vi "Advanced Serial Write and Read.vi"(4 "stop":bool, 5 "timeout (ms)":u32, 6 "baud rate":u32, 7 "VISA resource name":refnum<visa-resource-name>) -> (1 "gecorr. hoek":string, 2 "afstand":string, 3 "gecorrigeerde afstand":string)   [LabVIEW 8.6]
doc: "The Advanced Serial Read and Write example performs a Serial Port Read, a Serial Port Write, or a combination of these actions while setting some advanced serial features like buffer size, termination characters, and XON/XOFF flow control. The user selects the actions (read or write) on the front panel. If both are selected, the VI will write the data first, read the data and then close the VISA session that is opened to the port. \n\nThe parameters set for the serial port must match the parameters of the connected instrument or device. In this example, the bytes to read parameter specifies the number of bytes that the serial port reads. If there were more bytes at the port than the number specified in bytes to read, those bytes would not be read. Also, if you specify to read more bytes than the number of bytes actually read, you might receive a timeout error message.\n\nINSTRUCTIONS:\n1) Select the serial resource and configuration parameters (baud rate, data bits, parity, stop bits, flow control).\n2) Termination character can be enabled and set. Also, set the required input buffer size prior to running the example.\n3) Select the operations to be performed. \n4) Connect the serial port to your device. If no device is available, perform a loopback test by doing one of the following. Short pins 2 and 3 on a RS-232 cable or short pin 4 to pin 8 and pin 5 to pin 9 on a RS-485/422 cable. \n5) Run the VI to see the data read. (The \"read string\" will match the \"string to write\" if a loopback test was performed.)\n\nThis example exposes several advanced features that you may need for your application. Not all applications need all the features shown in this example. The input buffer size is likely an important setting that you want to control in your application. This example expands upon the flow control option for XON and XOFF, allowing the user to choose those control characters. The timeout parameter has been brought to the front panel so a user can specify the time period the VISA Read will wait for the number of bytes to read before timing out. Also, the user has several controls for the termination character, which is discussed later.\n\nNote that you can press the write and read buttons and change the bytes to read parameters on the fly, while the example is running. However, you must stop the example to change the other configuration parameters after the example has started running, and then run again.\n\nSet the I/O buffer size slightly higher the amount of data you expect to receive. This is very important for applications that don't use flow control, as you may lose characters if the receive buffer overflows.\n\nSetting the timeout period ensures that the operation returns with a timeout error if the operation cannot be performed in the specified time period. \n\nSome devices require a termination character in order to identify the end of command strings. Some devices send a termination character to signify the end of data to be read. \n\nThis example shows how you can end the Read operation once a termination character is detected in the buffer and/or append a termination character at the end of the Write data. To enable the Read to end on a termination character, use the VISA Configure Serial Port or use the VISA Properties Serial End Mode for Reads, Termination Character Enable, and Termination Character. To end the Write with a termination character, use the VISA Properties Serial End Mode for Writes, the Send End Enable, and Termination Character. In this example, the same termination character is used for both the Read and the Write. You can specify two different characters for your application, if desired.\n\nYour application may require specific characters for the XON/XOFF Flow Control. You can specify these characters with the VISA Properties Flow Control XOFF Character and Flow Control XON Character. Note that if the standard XON and XOFF characters are used, then decimal 17 and 19 are unavailable for data values. Remember that using flow control and setting an adequate buffer size allow you to prevent buffer overflows."
uses:
  <vilib>/Instr/_visa.llb/VISA Configure Serial Port (Instr).vi
panel:
  out "current time":timestamp
  out "current GPS time":timestamp
  in  "correctie voor hoek":dbl
  out "gemeten hoek":string
  out "concatenated string":string
  out "actual bytes read":u32
  in  "read":bool
  in  "bytes to read":u32
  out "read string":string
  in  "flow control":u16(ring) items=["None", "XON/XOFF", "RTS/CTS", "DTR/DSR"]
  in  "End write with termination character?":bool
  in  "Input\nbuffer size":u32
  in  "XOFF Character":u8 format="%.0x"
  in  "XON Character":u8 format="%.0x"
  in  "termination char\n(0xA = '\\n' = LF)":u8 format="%.0x"
  in  "End read on termination character?":bool
  in  "parity":u16(ring) items=["None", "Odd", "Even", "Mark", "Space"]
  in  "data bits":u16
  in  "stop bits":u16(ring) items=["1.0", "1.5", "2.0"]
  in  "write":bool
  in  "string to write":string
  # "On Windows/Linux, consider using the Instrument Driver Finder (Help>>Find Instrument Drivers) to search for an instrument driver for your instrument."
  # "Select the serial resource and the operations to be performed.  If all are selected, the VI will write the data first, read data and then close the VISA session that is opened to the port.  This VI will wait until the specified number of bytes is received at the port, until the timeout period is met, or until a termination character is received.  The default termination character in this example is the Line Feed ( ASCII 0xA, '\\n' ).  Also, set the required input buffer size prior to running the example.\nNote: The example loops until the STOP button is pressed."
  # "For additional information select File >> VI Properties >> Documentation"
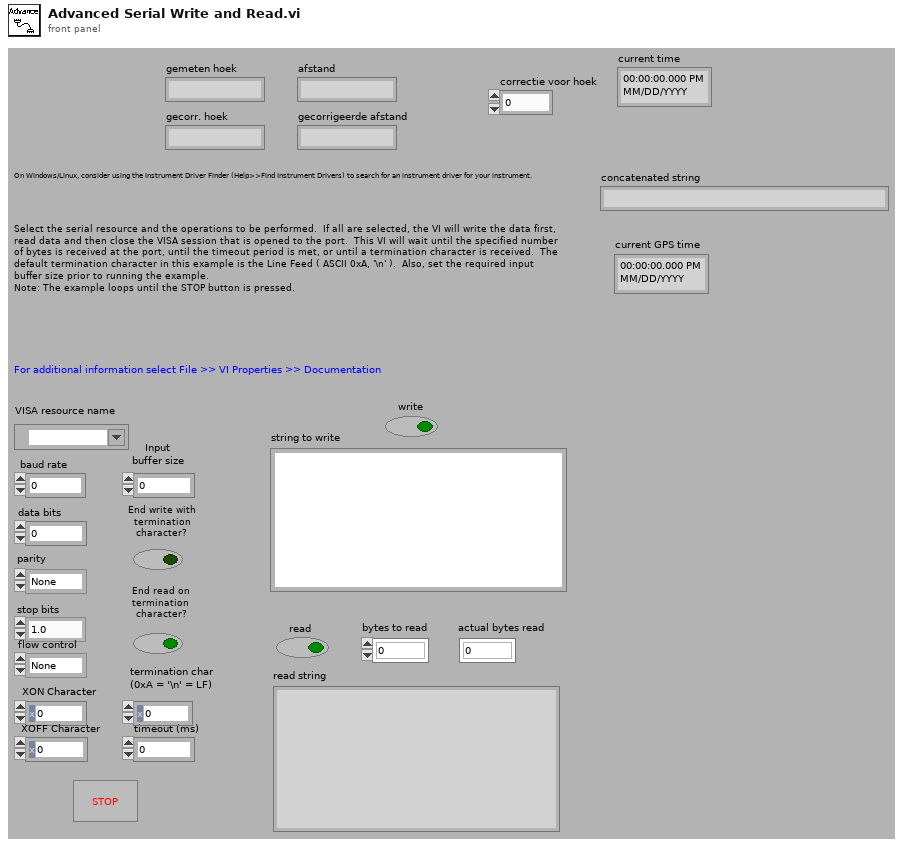
[diagram p1: front panel]
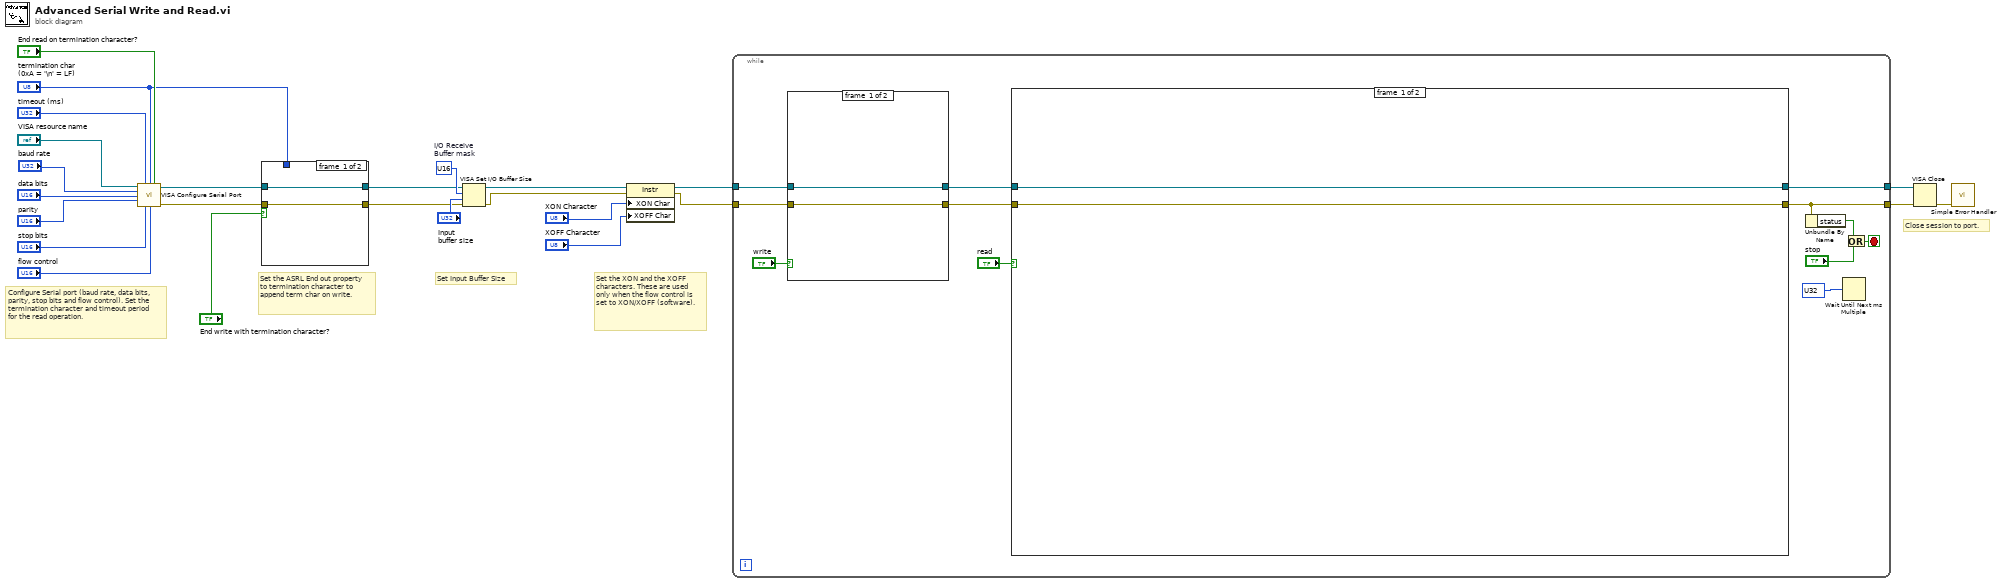
[diagram p0: block diagram]
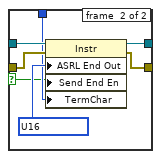
[diagram p2: hidden frame]
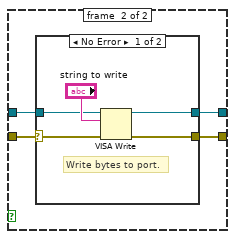
[diagram p3: hidden frame]
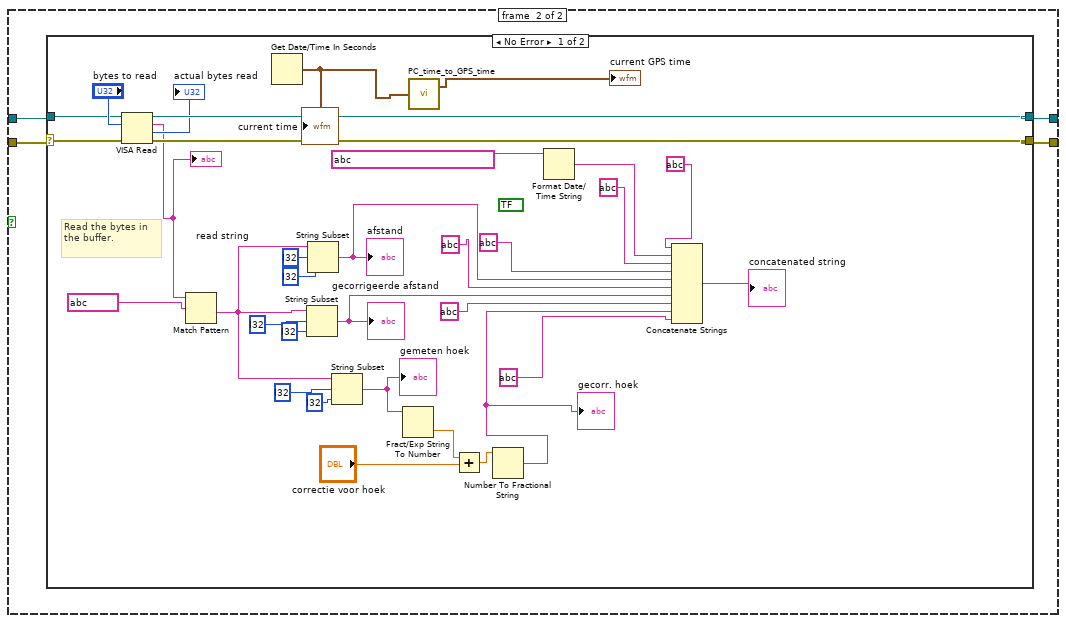
[diagram p5: hidden frame]
diagram:
  w18 = u16 ?  # I/O Receive Buffer mask
  # "Set the XON and the XOFF characters. These are used only when the flow control is set to XON/XOFF (software)."
  # "Configure Serial port (baud rate, data bits, parity, stop bits and flow control). Set the termination character and timeout period for the read operation."
  # "Set Input Buffer Size"
  # "Set the ASRL End out property to termination character to append term char on write."
  # "Close session to port."
  n1 = call-poly "VISA Configure Serial Port"("VISA resource name"="VISA resource name", "timeout (10sec)"="timeout (ms)", "termination char\n(0xA = '\\n' = LF)"="termination char\n(0xA = '\\n' = LF)", "Enable Termination\nChar (T)"="End read on termination character?", "baud rate (9600)"="baud rate", "data bits (8)"="data bits", "parity (0:none)"="parity", "stop bits (10: 1 bit)"="stop bits", "flow control (0:none)"="flow control") -> ("VISA resource name out"=w4:refnum<visa-resource-name>, "error out"=w7:errorcluster)  [unwired: 1 in, 4 out]
  n2 = case shown="True" "End write with termination character?" {
    selector: "End write with termination character?" -> [_ w28]
    tunnel: w4 -> [w26 w34]
    tunnel: w7 -> [w27 w33]
    tunnel: [w26 w32] -> w5
    tunnel: [w27 w31] -> w6
    tunnel: "termination char\n(0xA = '\\n' = LF)" -> [_ w29]
    frame #0 {
    }
    frame #1 {
      w30 = u16 ? items=["None", "LastBit", "TermChar", "Break"] ("Serial Settings:Serial End Mode for Writes")
      n3 = property class="Instr"(reference=w34, error in=w33, "ASRL End Out"=w30, "Send End En"=w28, "TermChar"=w29) -> (reference out=w32:refnum<visa-resource-name>, error out=w31:errorcluster)
    }
  }
  n4 = VISA Set I/O Buffer Size(VISA resource name=w5, mask (16)=w18, size (4096)="Input\nbuffer size", error in (no error)=w6) -> (VISA resource name out=w13:refnum<visa-resource-name>, error out=w12:errorcluster)
  n5 = property class="Instr"(reference=w13, error in=w12, "XON Char"="XON Character", "XOFF Char"="XOFF Character") -> (reference out=w3:refnum<visa-resource-name>, error out=w9:errorcluster)
  n6 = while {
    tunnel: w9 -> [w39]
    tunnel: w3 -> [w40]
    tunnel: [w38] -> w2
    tunnel: [w37] -> w1
    stop <- w36 stop-if-true
    n7 = case shown="True" "write" {
      tunnel: [w48 w52] -> w43
      tunnel: [w47 w51] -> w42
      tunnel: w40 -> [w48 w50]
      tunnel: w39 -> [w47 w49]
      frame #0 {
      }
      frame #1 {
        n8 = case shown="No Error" w49 {
          selector: w49 -> [w54 w59]
          tunnel: [w53 w58] -> w52
          tunnel: [w57 w59] -> w51
          tunnel: w50 -> [w55 w58]
          frame #0 {
            # "Write bytes to port."
            n9 = VISA Write(VISA resource name=w55, write buffer="string to write", error in (no error)=w54) -> (VISA resource name out=w53:refnum<visa-resource-name>, error out=w57:errorcluster)  [unwired: 1 out]
          }
          frame #1 {
          }
        }
      }
    }
    n10 = case shown="True" "read" {
      tunnel: w42 -> [w60 w63]
      tunnel: w43 -> [w61 w62]
      tunnel: [w60 w65] -> w37
      tunnel: [w61 w64] -> w38
      frame #0 {
      }
      frame #1 {
        n11 = case "Read bytes from port." shown="No Error" w63 {
          selector: w63 -> [w94 w99]
          tunnel: [w97 w99] -> w65
          tunnel: [w98 w100] -> w64
          tunnel: w62 -> [w95 w100]
          frame #0 {
            (unwired) bool ?
            # "Read the bytes in the buffer."
            n12 = VISA Read(VISA resource name=w95, byte count="bytes to read", error in (no error)=w94) -> (VISA resource name out=w98:refnum<visa-resource-name>, read buffer=w92:string, return count=→"actual bytes read":u32, error out=w97:errorcluster)
            "read string" <- w92
            n13 = Match Pattern(string=w92, regular expression=string ?) -> (after substring=w84:string)  [unwired: 1 in, 3 out]
            n14 = Get Date/Time In Seconds() -> (seconds since 1Jan1904=w71:timestamp)
            "current time" <- w71
            n15 = String Subset(string=w84, offset (0)=i32 ?, length (rest)=i32 ? ("length (rest)")) -> (substring=w80:string)
            "gecorrigeerde afstand" <- w80
            n16 = String Subset(string=w84, offset (0)=i32 ?, length (rest)=i32 ? ("length (rest)")) -> (substring=w82:string)
            "afstand" <- w82
            n17 = String Subset(string=w84, offset (0)=i32 ?, length (rest)=i32 ? ("length (rest)")) -> (substring=w77:string)
            "gemeten hoek" <- w77
            n18 = Fract/Exp String To Number(string=w77) -> (number=w75:dbl)  [unwired: 3 in, 1 out]
            n19 = call "PC_time_to_GPS_time.vi"("current PC time"=w71) -> ("current GPS time"=→"current GPS time":timestamp)  [unwired: 1 out]
            n20 = Add(x=w75, y="correctie voor hoek") -> (x+y=w74:dbl)
            n21 = Number To Fractional String(number=w74) -> (F-format string=w76:string)  [unwired: 3 in]
            "gecorr. hoek" <- w76
            n22 = Format Date/Time String(time format string (%c)=string ? ("%3u")) -> (date/time string=w67:string)  [unwired: 2 in]
            n23 = Concatenate Strings(string ?, w67, string ?, string ?, w82, string ?, w80, string ?, w76, string ?) -> (→"concatenated string":string)
          }
          frame #1 {
            # "Error occurred \nreading Bytes at \nSerial Port"
          }
        }
      }
    }
    n24 = Unbundle By Name(w37) -> ("status"=w44:bool)
    n25 = Wait Until Next ms Multiple(millisecond multiple=u32 ?) -> ()  [unwired: 1 out]
    n26 = Or(x=w44, y="stop") -> (x .or. y?=w36:bool)
  }
  n27 = VISA Close(VISA resource name=w2, error in (no error)=w1) -> (error out=w23:errorcluster)
  n28 = call <vilib>:"Simple Error Handler.vi"("error in (no error)"=w23) -> ()  [unwired: 1 in, 8 out]
